vi "AddressDecoder.vi"(1 "Address":u32) -> (0 "Address Cluster":T1={"Subsystem Id"=90, "Node Id"=1, "Component Id"=1})   [LabVIEW 2011]
uses:
  Address.ctl
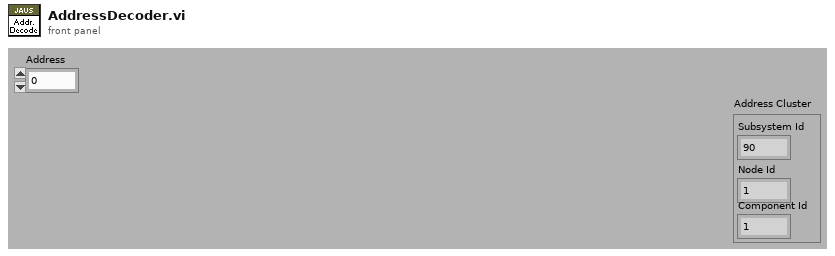
[diagram p1: front panel]
types:
  T1 = typedef "Address.ctl" = cluster{"Subsystem Id":u16, "Node Id":u8, "Component Id":u8}
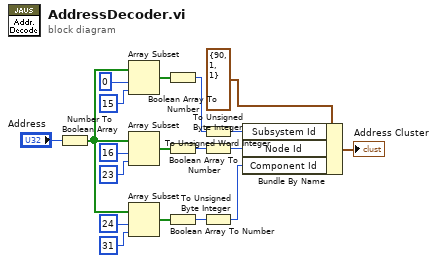
[diagram p0: block diagram]
diagram:
  n1 = Number To Boolean Array(number="Address") -> (Boolean array=w13:bool[])
  n2 = Array Subset(array=w13, index=0, length=15) -> (w16:bool[])
  n3 = Array Subset(array=w13, index=16, length=23) -> (w10:bool[])
  n4 = Array Subset(array=w13, index=24, length=31) -> (w9:bool[])
  n5 = Boolean Array To Number(Boolean array=w16) -> (number=w8:u32)
  n6 = Boolean Array To Number(Boolean array=w10) -> (number=w7:u32)
  n7 = Boolean Array To Number(Boolean array=w9) -> (number=w6:u32)
  n8 = To Unsigned Word Integer(number=w8) -> (unsigned 16bit integer=w3:u16)
  n9 = To Unsigned Byte Integer(number=w7) -> (unsigned 8bit integer=w2:u8)
  n10 = To Unsigned Byte Integer(number=w6) -> (unsigned 8bit integer=w1:u8)
  n11 = Bundle By Name(cluster=T1 {"Subsystem Id"=90, "Node Id"=1, "Component Id"=1} ("Address Cluster"), "Subsystem Id"=w3, "Node Id"=w2, "Component Id"=w1) -> (→"Address Cluster":T1)
